vi "To String.Integer.Decimal.U64.vi"(1 "value":u64) -> (0 "value as string":string)   [LabVIEW 2016, in "Memory Manager.lvlib" / "Static Error Handling.lvlib"]
doc: "Converts the provided <B>value</B> into a decimal-formatted string."
uses:
  Static Error Handling.lvlib
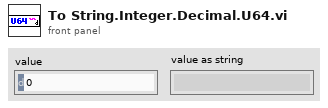
[diagram p1: front panel]
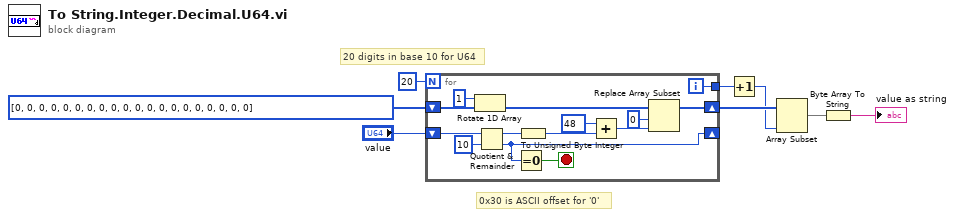
[diagram p0: block diagram]
diagram:
  # "0x30 is ASCII offset for '0'"
  # "20 digits in base 10 for U64"
  n1 = for {
    N: 20 -> [_]
    shift-right: [w21] -> w4
    shift-left: u8[] [0, 0, 0, 0, 0, 0, 0, 0, 0, 0, 0, 0, 0, 0, 0, 0, 0, 0, 0, 0] -> [w13]
    shift-right: [w16] -> _
    shift-left: "value" -> [w18]
    tunnel: [w10] -> w2
    i -> [w10]
    stop <- w15 stop-if-true
    n2 = Rotate 1D Array(1:w13, 2:1 ("n")) -> (0:w12:u8[])
    n3 = Quotient & Remainder(x=w18, y=u64 10) -> (x-y*floor(x/y)=w17:u64, floor(x/y)=w16:u64)
    n4 = Equal To 0?(x=w16) -> (x = 0?=w15:bool)
    n5 = To Unsigned Byte Integer(number=w17) -> (unsigned 8bit integer=w9:u8)
    n6 = Add(x=u8 48 ("y"), y=w9) -> (x+y=w22:u8)
    n7 = Replace Array Subset(array=w12, new element=w22, index=0) -> (w21:u8[])
  }
  n8 = Increment(x=w2) -> (x+1=w1:i32)
  n9 = Array Subset(array=w4, length=w1) -> (w3:u8[])  [unwired: 1 in]
  n10 = Byte Array To String(unsigned byte array=w3) -> (string=→"value as string":string)
